vi "Set SLSC Switch Topology.vi"(8 "error in":errorcluster, 10 "topology":string, 11 "slsc switch custom device in":T1 format="%.0x") -> (0 "error out":errorcluster, 3 "slsc switch custom device out":T1 format="%.0x")   [LabVIEW 2017, in "SLSC Switch Scripting.lvlib"]
doc: "Sets the topology for the SLSC Switch custom device."
uses:
  SLSC Switch Scripting.lvlib
  <vilib>/NI Veristand/Custom Device API/Custom Device Item Ref.ctl
  <vilib>/NI Veristand/Custom Device API/Custom Device API.lvlib
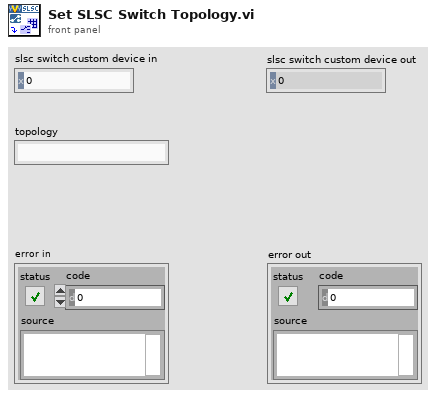
[diagram p1: front panel]
types:
  T1 = typedef "Custom Device API.lvlib/Custom Device Item Ref.ctl" = u64
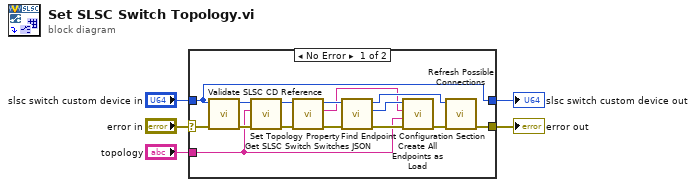
[diagram p0: block diagram]
diagram:
  n1 = case shown="No Error" "error in" {
    selector: "error in" -> [w7 w22]
    tunnel: "topology" -> [w6 _]
    tunnel: [w13 w22] -> w5
    tunnel: "slsc switch custom device in" -> [w8 w21]
    tunnel: [w8 w21] -> w2
    frame No Error {
      n2 = call "Validate SLSC CD Reference.vi"("error in"=w7, "slsc switch custom device in"=w8) -> ("error out"=w9:errorcluster, "slsc switch custom device out"=w10:T1)  [unwired: 8 in]
      n3 = call "Set Topology Property.vi"("error in"=w9, "topology"=w6, "slsc switch custom device in"=w10) -> ("error out"=w12:errorcluster, "slsc switch custom device out"=w11:T1)  [unwired: 7 in]
      n4 = call "Get SLSC Switch Switches JSON.vi"("error in"=w12, "slsc switch custom device in"=w11) -> ("error out"=w17:errorcluster, "switches json"=w15:string, "slsc switch custom device out"=w16:T1)  [unwired: 7 in]
      n5 = call "Find Endpoint Configuration Section.vi"("error in"=w17, "slsc switch custom device in"=w16) -> ("error out"=w18:errorcluster, "endpoint configuration"=w19:T1, "slsc switch custom device out"=w20:T1)  [unwired: 7 in]
      n6 = call "Create All Endpoints as Load.vi"("error in"=w18, "topology"=w6, "switches json"=w15, "endpoint configuration in"=w19) -> ("error out"=w14:errorcluster)  [unwired: 6 in, 1 out]
      n7 = call "Refresh Possible Connections.vi"("error in"=w14, "slsc switch custom device in"=w20) -> ("error out"=w13:errorcluster)  [unwired: 8 in, 1 out]
    }
    frame Error {
    }
  }
  "error out" <- w5
  "slsc switch custom device out" <- w2
